vi "Data Packaging Loop deprecated.vi"(8 "error in（no error）":errorcluster caption="错误输入（无错误）", 9 "channel info array":T2(array[cluster]) caption="通道信息数组", 10 "channel data queue":refnum<queue> caption="通道数据队列", 11 "Message Queues":T1 caption="消息队列") -> (0 "error out":errorcluster caption="错误输出")   [LabVIEW 2015]
uses:
  Globals/Global - Monitoring Variables.vi
  <vilib>/Waveform/WDTOps.llb/WDT Index Channel DBL.vi
  <vilib>/Waveform/WDTOps.llb/WDT Get Final Time Value DBL.vi
  <vilib>/Waveform/WDTOps.llb/WDT Append Waveforms DBL.vi
  <vilib>/Waveform/WDTOps.llb/WDT Waveform Duration DBL.vi
  support/Message Queue/Message Queue.lvlib
  Globals/Global - All RT Loop Stop.vi
  support/Message Queue/Message Cluster.ctl
  support/Message Queue/All Real-Time Message Queues.ctl
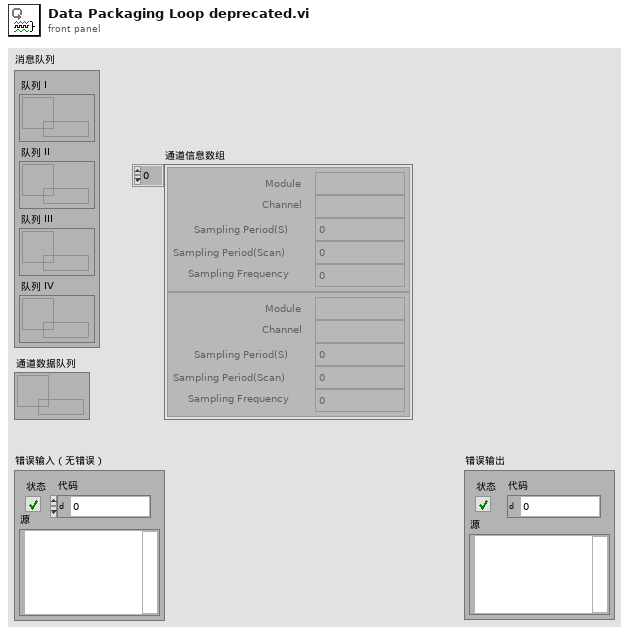
[diagram p1: front panel]
types:
  T1 = typedef "Message Queue.lvlib/All Real-Time Message Queues.ctl" = cluster{"Queue I":refnum<queue>, "Queue II":refnum<queue>, "Queue III":refnum<queue>, "Queue IV":refnum<queue>}
  T2 = cluster{"Module":string, "Channel":string, "Sampling Period(S)":dbl, "Sampling Period(Scan)":i64, "Sampling Frequency":i64}[]
  T3 = enum16{"Initialize", "Acquire Data", "Create Waveform", "Append Waveform", "Send Waveform"}
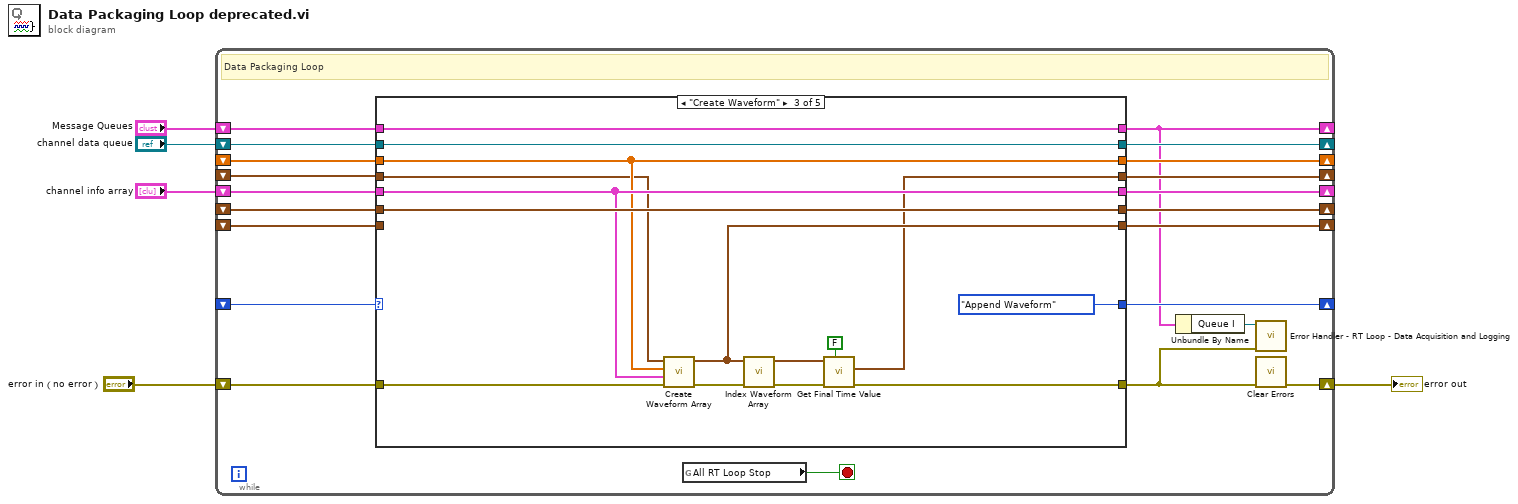
[diagram p0: block diagram]
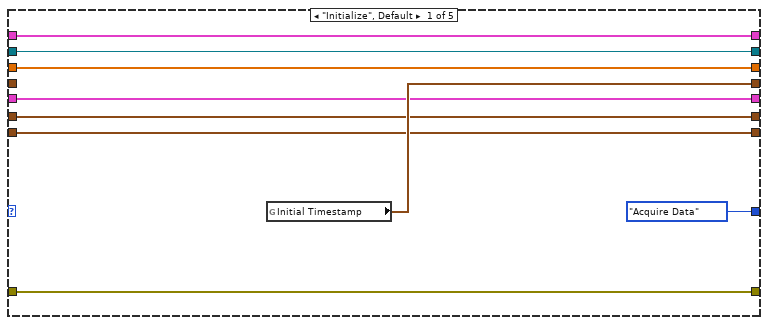
[diagram p2: hidden frame]
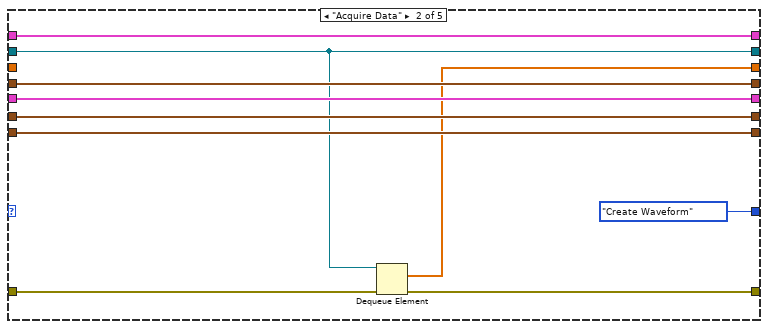
[diagram p3: hidden frame]
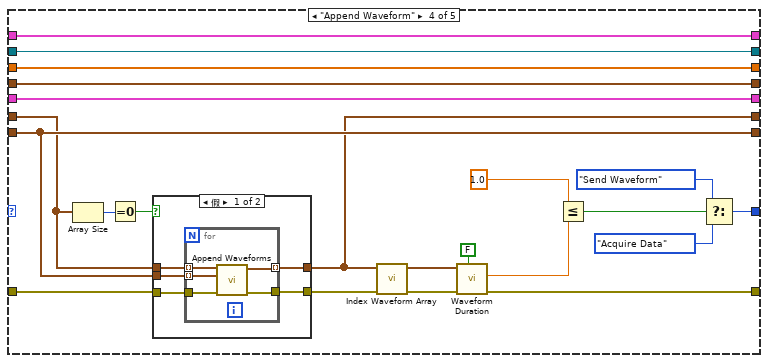
[diagram p4: hidden frame]
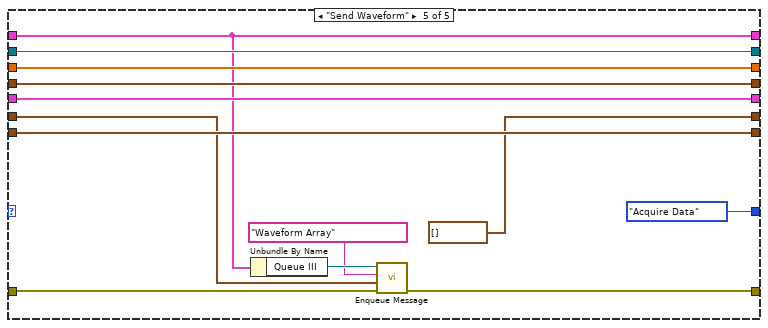
[diagram p6: hidden frame]
diagram:
  n1 = while {
    shift-right: [w26] -> _
    shift-left: _ -> [w25]
    shift-right: [w24] -> _
    shift-left: _ -> [w23]
    shift-right: [w17] -> _
    shift-left: _ -> [w18]
    shift-right: [w6] -> _
    shift-left: "Message Queues" -> [w16]
    shift-right: [w15] -> _
    shift-left: _ -> [w14]
    shift-right: [w13] -> w1
    shift-left: "error in（no error）" -> [w21]
    shift-right: [w10] -> _
    shift-left: "channel data queue" -> [w22]
    shift-right: [w9] -> _
    shift-left: "channel info array" -> [w19]
    shift-right: [w8] -> _
    shift-left: _ -> [w7]
    stop <- w20 stop-if-true
    # "Data Packaging Loop"
    n2 = case shown="\"Create Waveform\"" w18 {
      tunnel: [w29 w45 w60 w70 waveform(dbl)[] []] -> w26
      tunnel: w25 -> [w29 w45 w60 w74 w96]
      tunnel: [w34 w43 w46 w67 w106] -> w24
      tunnel: w23 -> [_ w43 w47 w67 w106]
      tunnel: w19 -> [w30 w39 w56 w76 w99]
      tunnel: w22 -> [w32 w37 w58 w78 w101]
      tunnel: w21 -> [w35 w41 w57 w77 w105]
      tunnel: [w35 w42 w48 w68 w104] -> w12
      tunnel: [T3."Acquire Data" T3."Create Waveform" T3."Append Waveform" w65 T3."Acquire Data"] -> w17
      tunnel: w16 -> [w33 w40 w59 w79 w97]
      tunnel: [w33 w40 w59 w79 w97] -> w6
      tunnel: [w31 w38 w55 w75 w100] -> w15
      tunnel: w14 -> [w31 _ w55 w75 w100]
      tunnel: [w32 w37 w58 w78 w101] -> w10
      tunnel: [w30 w39 w56 w76 w99] -> w9
      tunnel: [w28 w44 w52 w82 w98] -> w8
      tunnel: w7 -> [w28 w44 _ w82 w98]
      frame "Initialize", Default {
        n3 = global read "Global - Monitoring Variables.vi" "Initial Timestamp"() -> (w34:timestamp)
      }
      frame "Acquire Data" {
        n4 = Dequeue Element(queue=w37, error in (no error)=w41) -> (element=w38:dbl[], error out=w42:errorcluster)  [unwired: 1 in, 2 out]
      }
      frame "Create Waveform" {
        n5 = call "Create Waveform Array.vi"("error in (no error)"=w57, "samples to write"=w56, "sampling period (s)"=w55, "Timestamp"=w47) -> ("error out"=w53:errorcluster, "Waveform Array"=w52:waveform(dbl)[])  [unwired: 6 in]
        n6 = call-poly <vilib>:"Index Waveform Array.vi"("error in (no error)"=w53, "waveform array"=w52) -> ("error out"=w51:errorcluster, "waveform"=w50:waveform(dbl))  [unwired: 8 in]
        n7 = call-poly <vilib>:"Get Final Time Value.vi"("open interval? (T)"=FALSE, "error in (no error)"=w51, "waveform in"=w50) -> ("error out"=w48:errorcluster, "tf"=w46:timestamp)  [unwired: 6 in, 1 out]
      }
      frame "Append Waveform" {
        n8 = Array Size(array=w74) -> (size(s)=w81:i32)
        n9 = Equal To 0?(x=w81) -> (x = 0?=w80:bool)
        n10 = case shown="假" w80 {
          tunnel: w77 -> [w87 w93]
          tunnel: [w86 w93] -> w72
          tunnel: w82 -> [w85 w94]
          tunnel: [w84 w94] -> w70
          tunnel: w74 -> [w83 _]
          frame False {
            n11 = for {
              tunnel: w87 -> [w92]
              tunnel: [w91] -> w86
              tunnel: w85 -> [w90] mode=indexing
              tunnel: w83 -> [w89] mode=indexing
              tunnel: [w88] -> w84 mode=indexing
              n12 = call-poly <vilib>:"Append Waveforms.vi"("error in (no error)"=w92, "waveform B"=w90, "waveform A"=w89) -> ("error out"=w91:errorcluster, "waveform out"=w88:waveform(dbl))  [unwired: 7 in]
            }
          }
          frame True {
          }
        }
        n13 = call-poly <vilib>:"Index Waveform Array.vi"("error in (no error)"=w72, "waveform array"=w70) -> ("error out"=w71:errorcluster, "waveform"=w73:waveform(dbl))  [unwired: 8 in]
        n14 = call-poly <vilib>:"Waveform Duration.vi"("open interval? (T)"=FALSE, "error in (no error)"=w71, "waveform in"=w73) -> ("error out"=w68:errorcluster, "duration"=w69:dbl)  [unwired: 6 in, 1 out]
        n15 = Less Or Equal?(x=1.0, y=w69) -> (x <= y?=w66:bool)
        n16 = Select(t=T3."Send Waveform", s=w66, f=T3."Acquire Data") -> (s? t:f=w65:T3)
      }
      frame "Send Waveform" {
        n17 = Unbundle By Name(w97) -> ("Queue III"=w103:refnum<queue>)
        n18 = call "Enqueue Message.vi"("error in (no error)"=w105, "Message Data"=w96, "Message"="Waveform Array", "Message Queue"=w103) -> ("error out"=w104:errorcluster)  [unwired: 6 in, 1 out]
      }
    }
    n19 = global read "Global - All RT Loop Stop.vi" "All RT Loop Stop"() -> (w20:bool)
    n20 = Unbundle By Name(w6) -> ("Queue I"=w11:refnum<queue>)
    n21 = call "Error Handler - RT Loop - Data Acquisition and Logging.vi"("error in (no error)"=w12, "Message Queue"=w11) -> ()  [unwired: 9 in, 1 out]
    n22 = call <vilib>:"Clear Errors.vi"("error in (no error)"=w12) -> ("error out"=w13:errorcluster)  [unwired: 5 in, 1 out]
  }
  "error out" <- w1
